vi "Set_Act_Voltage_Meas_Resistance.vi"(0 "Keithley 2450 SMU":refnum<visa-resource-name>="GPIB0::9::INSTR", 1 "Keithley 2400 PULL-UP Actuator PS":refnum<visa-resource-name>="GPIB0::3::INSTR", 3 "4-Wire Measurement Delay (s)":dbl=0.001, 4 "Keithley 2400 PULL-DN Actuator PS":refnum<visa-resource-name>="GPIB0::3::INSTR", 5 "Error In":errorcluster, 6 "Pull-Up Actuation Voltage (V)":dbl, 7 "Forced Current (A)":dbl, 8 "Current Limit Pull-Up(A)":dbl=0.1, 9 "Compliance Limit (A)":dbl, 10 "Current Limit Pull-DN (A)":dbl=0.1, 11 "SENSE VLIM":dbl, 12 "Pull-Down Actuation Voltage (V)":dbl) -> (15 "Measured Resistance (Ohms)":string="0", 17 "Meas Forced Current (A)":string, 19 "Error Out":errorcluster)   [LabVIEW 2017]
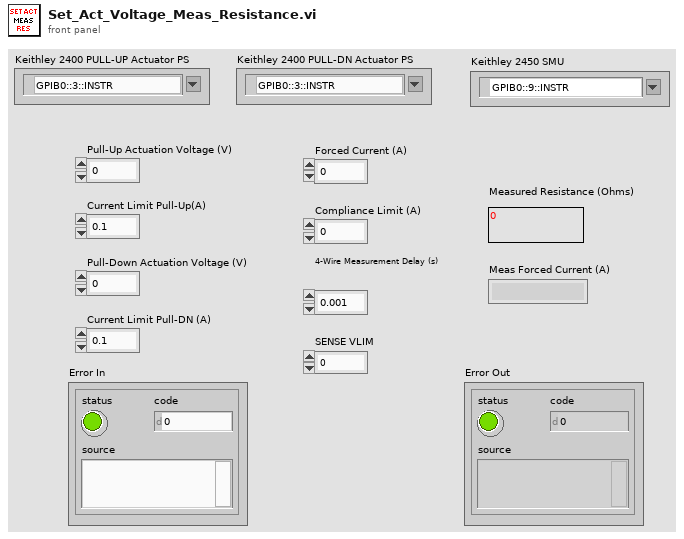
[diagram p1: front panel]
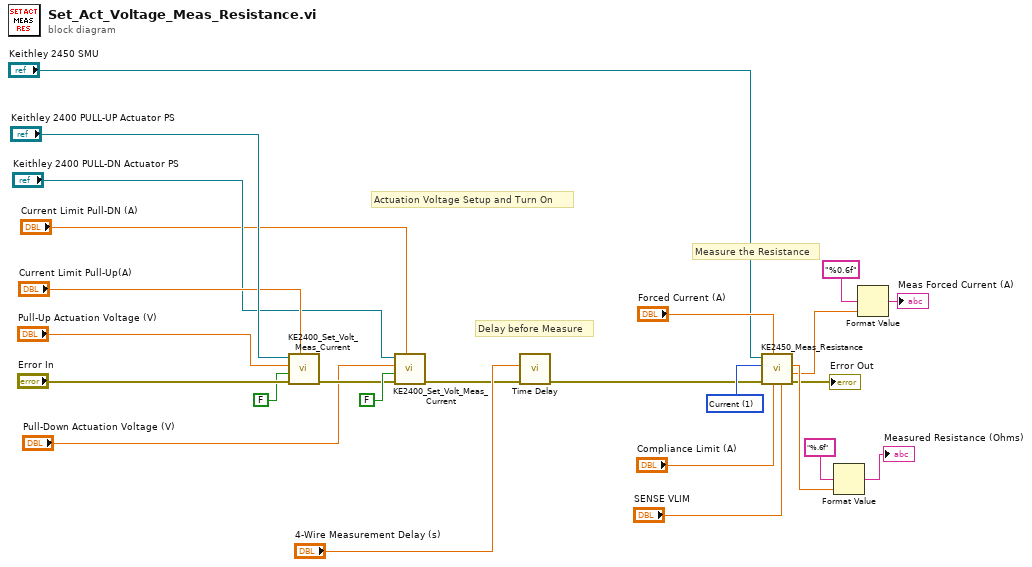
[diagram p0: block diagram]
diagram:
  w24 = u16 1 items=["Voltage", "Current"] ("Source Mode  (0: Voltage)")
  # "Actuation Voltage Setup and Turn On"
  # "Delay before Measure"
  # "Measure the Resistance"
  n1 = call "KE2400_Set_Volt_Meas_Current.vi"("Compliance  Level (0.1)"="Current Limit Pull-Up(A)", "error in (no error)"="Error In", "Enable Remote Sensing (T: Enable)"=FALSE, "Output Level (0)"="Pull-Up Actuation Voltage (V)", "VISA resource name"="Keithley 2400 PULL-UP Actuator PS") -> ("error out"=w10:errorcluster)  [unwired: 4 in, 2 out]
  n2 = call "KE2400_Set_Volt_Meas_Current.vi"("Compliance  Level (0.1)"="Current Limit Pull-DN (A)", "error in (no error)"=w10, "Enable Remote Sensing (T: Enable)"=FALSE, "Output Level (0)"="Pull-Down Actuation Voltage (V)", "VISA resource name"="Keithley 2400 PULL-DN Actuator PS") -> ("error out"=w13:errorcluster)  [unwired: 4 in, 2 out]
  n3 = call "Time Delay"("error in (no error)"=w13, "Delay Time (s)"="4-Wire Measurement Delay (s)") -> ("error out"=w15:errorcluster)  [unwired: 9 in]
  n4 = call "KE2450_Meas_Resistance.vi"("SENSE VLIM"="SENSE VLIM", "Compliance Level (0.1)"="Compliance Limit (A)", "Output Level (0)"="Forced Current (A)", "error in (no error)"=w15, "Source Mode  (0: Voltage)"=w24, "VISA resource name"="Keithley 2450 SMU") -> ("error out"=→"Error Out":errorcluster, "Current Level Out (A)"=w2:dbl, "Resistance (ohm)"=w20:dbl)  [unwired: 3 in]
  n5 = Format Value(format string="%.6f", value (0)=w20) -> (output string=→"Measured Resistance (Ohms)":string)  [unwired: 1 in]
  n6 = Format Value(format string="%0.6f", value (0)=w2) -> (output string=→"Meas Forced Current (A)":string)  [unwired: 1 in]
